vi "TEST Object Manual Bounds (Show Hide).vi"() -> ()   [LabVIEW 2013, in "IObject.lvclass"]
uses:
  IObject.lvclass
  <vilib>/Utility/miscctls.llb/LVRectTypeDef.ctl
  IContainer/Viewport/Viewport.lvclass
  Object/Object.lvclass
panel:
  in  "OK Button 4":bool
  in  "OK Button 3":bool
  in  "OK Button 2":bool
  in  "Bounds":T1={"Left"=100, "Top"=10, "Right"=400, "Bottom"=250}
  in  "OK Button 1":bool
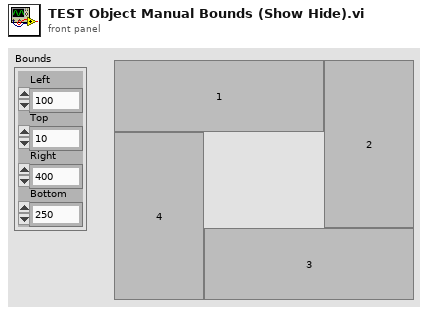
[diagram p1: front panel]
types:
  T1 = typedef "LVRectTypeDef.ctl" = cluster{"Left":i16, "Top":i16, "Right":i16, "Bottom":i16}
  T2 = cluster{"Left":dbl, "Top":dbl, "Right":dbl, "Bottom":dbl}[]
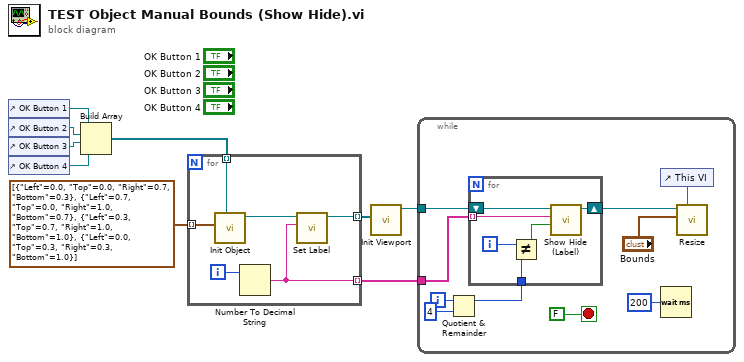
[diagram p0: block diagram]
diagram:
  n1 = control-ref of="OK Button 1"() -> (w9:refnum<vi>)
  n2 = control-ref of="OK Button 2"() -> (w8:refnum<vi>)
  n3 = control-ref of="OK Button 3"() -> (w7:refnum<vi>)
  n4 = control-ref of="OK Button 4"() -> (w6:refnum<vi>)
  n5 = Build Array(w9, w8, w7, w6) -> (w5:refnum<vi>[])
  n6 = for {
    tunnel: T2 [{"Left"=0.0, "Top"=0.0, "Right"=0.7, "Bottom"=0.3}, {"Left"=0.7, "Top"=0.0, "Right"=1.0, "Bottom"=0.7}, {"Left"=0.3, "Top"=0.7, "Right"=1.0, "Bottom"=1.0}, {"Left"=0.0, "Top"=0.3, "Right"=0.3, "Bottom"=1.0}] -> [w14] mode=indexing
    tunnel: w5 -> [w13] mode=indexing
    tunnel: [w12] -> w3 mode=indexing
    tunnel: [w10] -> w1 mode=indexing
    i -> [w11]
    n7 = call "Init Object.vi"("GObj Refnum"=w13, "A [0, 0, 1, 1]"=w14) -> ("MMI Scaling out"=w15:refnum<class "Object.lvclass">)  [unwired: 8 in, 1 out]
    n8 = Number To Decimal String(number=w11) -> (decimal integer string=w10:string)  [unwired: 1 in]
    n9 = call "Set Label.vi"("Label"=w10, "MMI Scaling in"=w15) -> ("MMI Scaling out"=w12:refnum<class "Object.lvclass">)  [unwired: 8 in, 1 out]
  }
  n10 = call "Init Viewport.vi"("Items"=w3) -> ("Viewport out"=w2:refnum<class "Viewport.lvclass">)  [unwired: 9 in, 1 out]
  n11 = while {
    tunnel: w2 -> [w25]
    tunnel: w1 -> [w22]
    i -> [w24]
    stop <- FALSE stop-if-true
    n12 = Quotient & Remainder(x=w24, y=4) -> (x-y*floor(x/y)=w21:i32)  [unwired: 1 out]
    n13 = for {
      tunnel: w22 -> [w30] mode=indexing
      shift-right: [w29] -> w17
      shift-left: w25 -> [w31]
      tunnel: w21 -> [w27]
      i -> [w28]
      n14 = Not Equal?(x=w28, y=w27) -> (x != y?=w26:bool)
      n15 = call-dynamic "Show Hide (Label).vi"("Show? [T]"=w26, "Label"=w30, "MMI Scaling in"=w31) -> ("MMI Scaling out"=w29:refnum<class "Viewport.lvclass">)  [unwired: 6 in, 2 out]
    }
    n16 = control-ref of="This VI"() -> (w18:refnum<vi>)
    n17 = Wait (ms)(milliseconds to wait=u32 200) -> ()  [unwired: 1 out]
    n18 = call-dynamic "Resize.vi"("VI Refnum"=w18, "Bounds"="Bounds", "MMI Scaling in"=w17) -> ()  [unwired: 6 in, 3 out]
  }
